vi "qVLS.vi"(0 "System no.":i32=1 min=1 max=4 step=1, 5 "error in":errorcluster) -> (14 "Velocity":dbl format="%.6f", 19 "error out":errorcluster)   [LabVIEW 2020]
doc: "Returns platform velocity setting.\n\nC-887, F-206, M-8X0: Only for GCS syntax version = GCS 2.0 or higher (check with CSV?.vi. If CSV?.vi is not supported, syntax version is GCS 1.0)."
panel:
  # "Returns platform velocity setting."
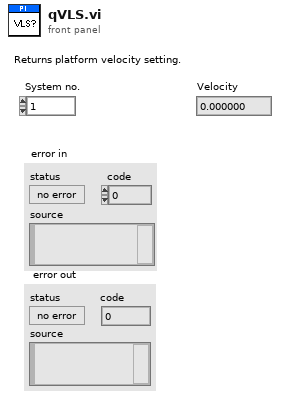
[diagram p1: front panel]
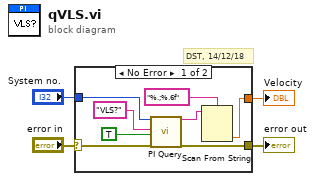
[diagram p0: block diagram]
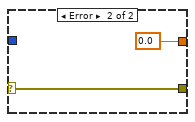
[diagram p2: hidden frame]
diagram:
  # "DST, 14/12/18"
  n1 = case shown="No Error" "error in" {
    selector: "error in" -> [w7 w13]
    tunnel: [w5 w13] -> w4
    tunnel: "System no." -> [w11 _]
    tunnel: [w8 0.0 ("Numeric")] -> w2
    frame No Error {
      n2 = call "PI Query.vi"("System no."=w11, "String to send"="VLS?", "Attach termination char.?"=TRUE ("Attach Linefeed?"), "error in"=w7) -> ("String read"=w6:string, "error out"=w5:errorcluster)  [unwired: 3 in, 11 out]
      n3 = Scan From String(format string="%.;%.6f" ("Format String"), input string=w6) -> (output 1=w8:dbl)  [unwired: 2 in, 4 out]
    }
    frame Error {
    }
  }
  "error out" <- w4
  "Velocity" <- w2
